vi "Rotate To Angle.vi"(0 "Angle (degrees)":dbl) -> ()   [LabVIEW 2015]
uses:
  navX Library v2/navX Library v2.lvlib
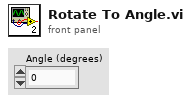
[diagram p1: front panel]
types:
  T1 = typedef "navX Library v2.lvlib/Z900_navX_DeviceTypeDef.ctl" = cluster{"Interface":cluster{"Protocol":T2, "Update Rate (4Hz-60Hz)":u8, "navX Open TypeDef":variant}, "Notify Packet":refnum<notifier>, "Loop VI Refnum":refnum<vi>, "Ready to Close Occurrence Refnum":refnum<k4>}
  T2 = typedef "navX Library v2.lvlib/Z900_navX_ProtocolTypeDef.ctl" = enum16{"SERIAL", "I2C", "SPI"}
  T3 = cluster{"Yaw":dbl, "Roll":dbl, "Pitch":dbl, "Heading":dbl, "Fused Heading":dbl}
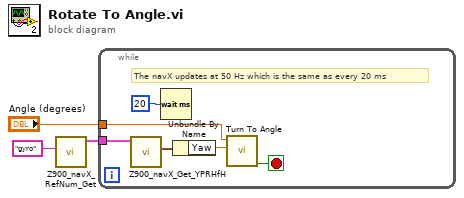
[diagram p0: block diagram]
diagram:
  n1 = call "Z900_navX_RefNum_Get.vi"("refnum name"="gyro") -> ("navX Device"=w1:T1)  [unwired: 9 in, 1 out]
  n2 = while {
    tunnel: w1 -> [w6]
    tunnel: "Angle (degrees)" -> [w5]
    stop <- w7 stop-if-true
    # "The navX updates at 50 Hz which is the same as every 20 ms"
    n3 = call "Z900_navX_Get_YPRHfH.vi"("navX Device"=w6) -> ("YRPHfH"=w9:T3)  [unwired: 7 in, 3 out]
    n4 = Wait (ms)(milliseconds to wait=u32 20) -> ()  [unwired: 1 out]
    n5 = Unbundle By Name(w9) -> ("Yaw"=w8:dbl)
    n6 = call "Turn To Angle.vi"("Current Angle"=w8, "Target Angle"=w5) -> ("Finished"=w7:bool)  [unwired: 9 in]
  }
